vi "Lab Panel V4.83.vi"() -> ()   [LabVIEW 2013] (continued)
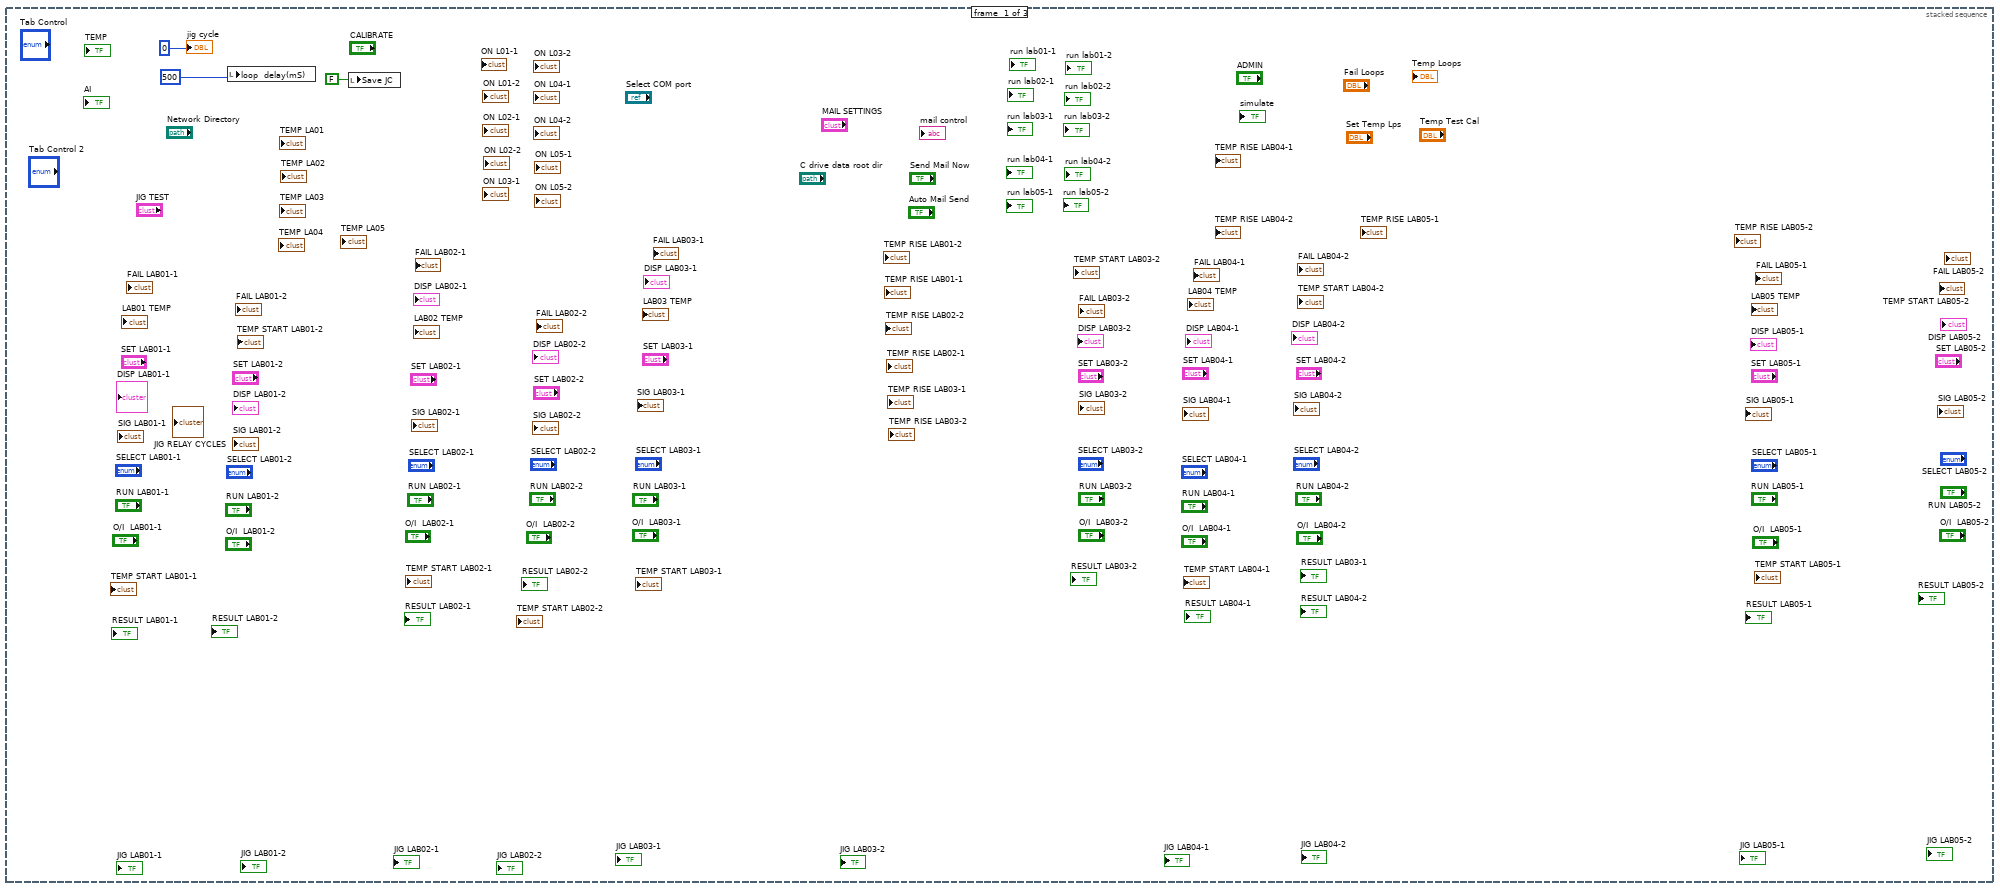
[diagram p2: hidden frame]
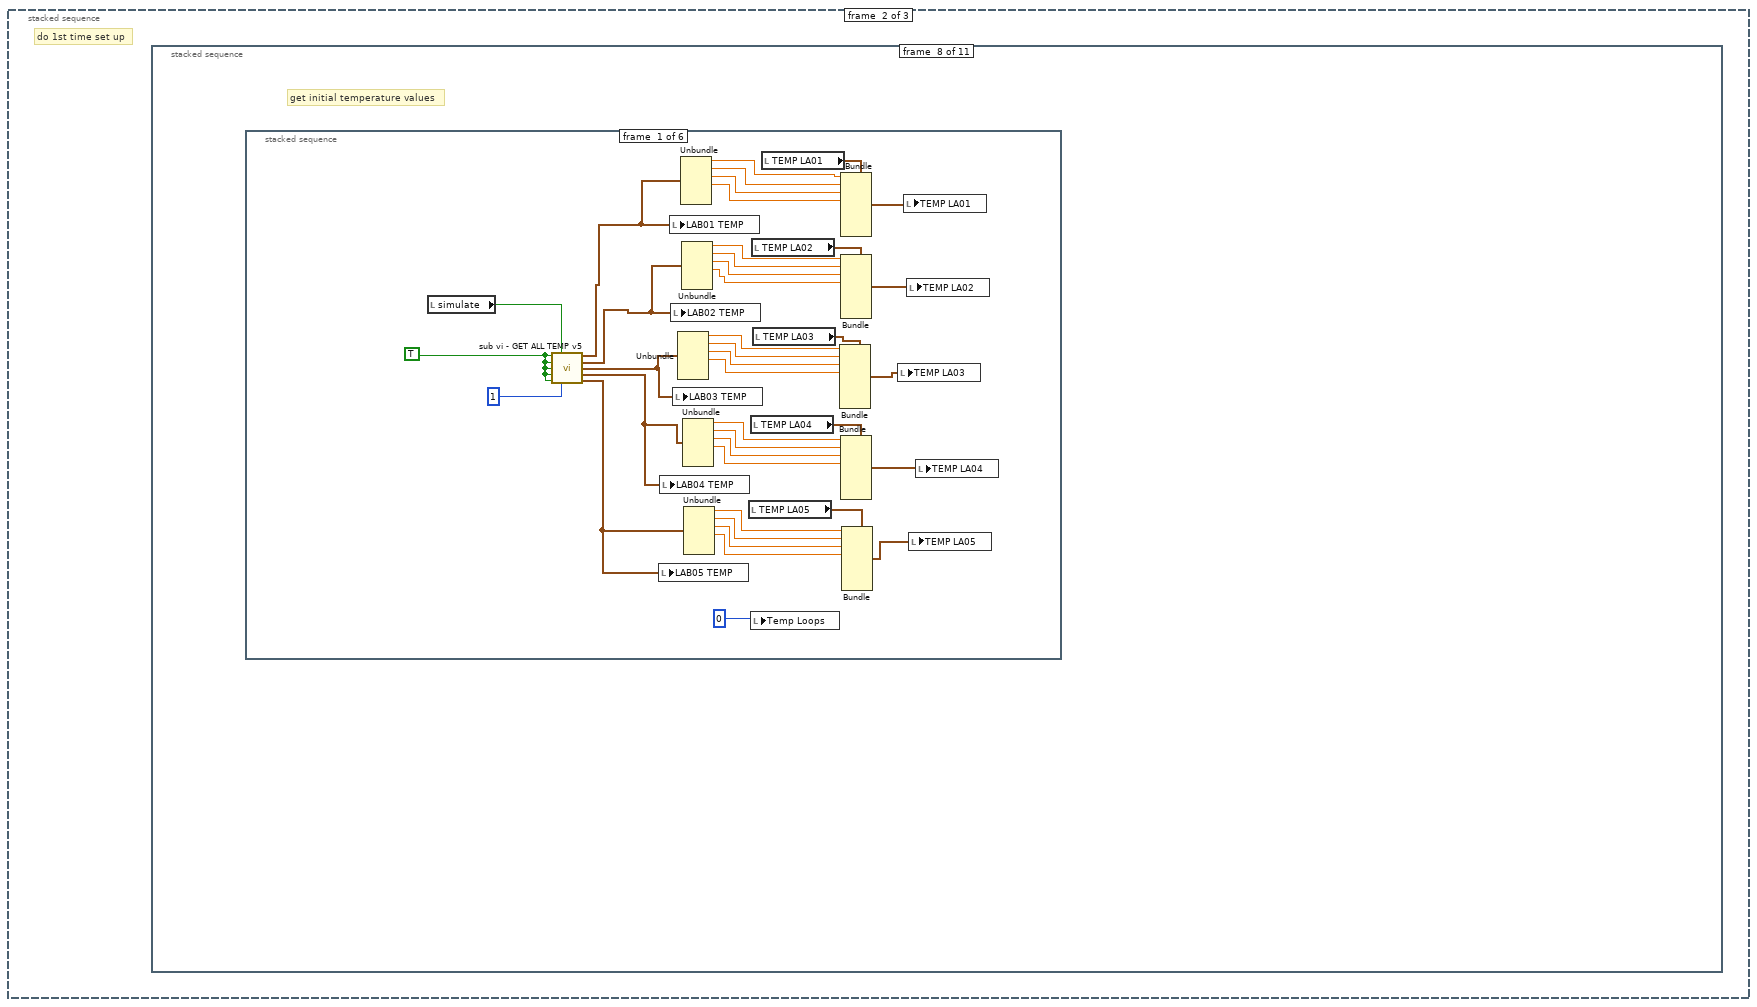
[diagram p3: hidden frame]
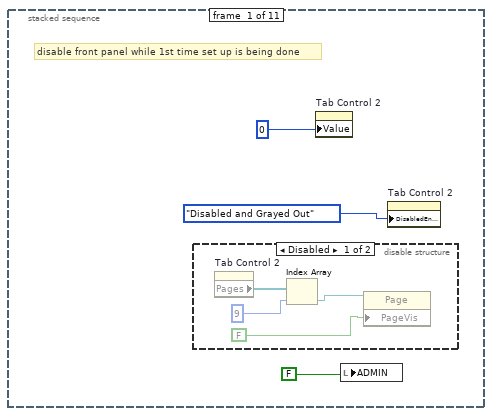
[diagram p4: hidden frame]
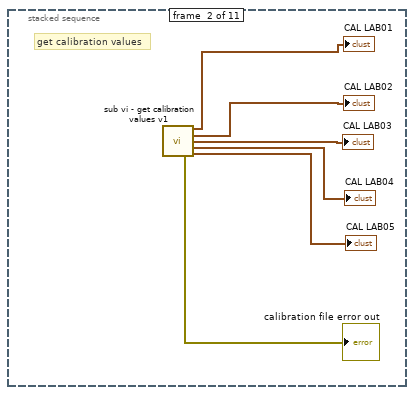
[diagram p6: hidden frame]
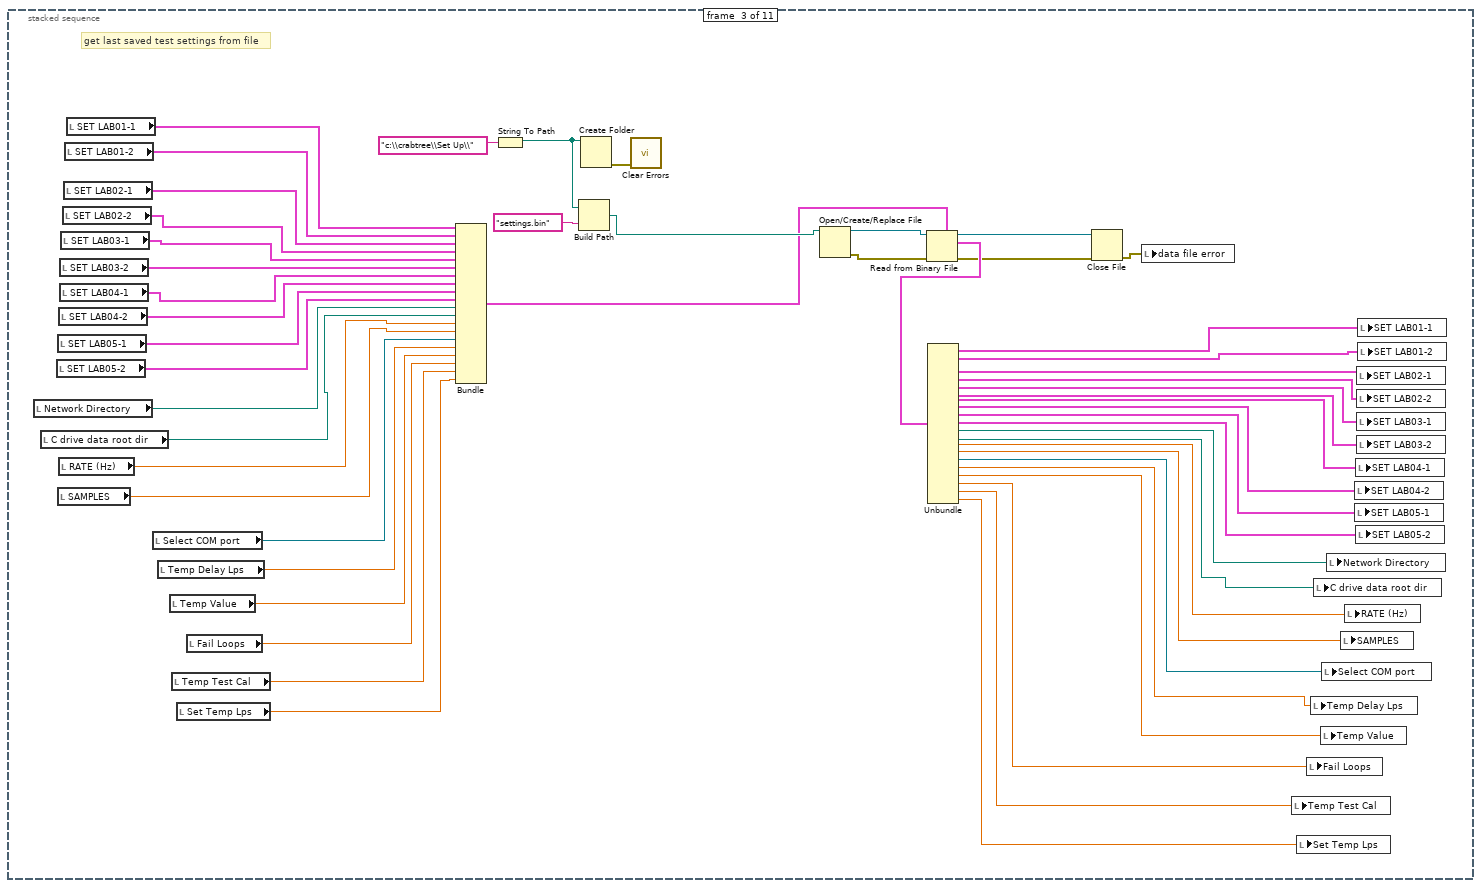
[diagram p7: hidden frame]
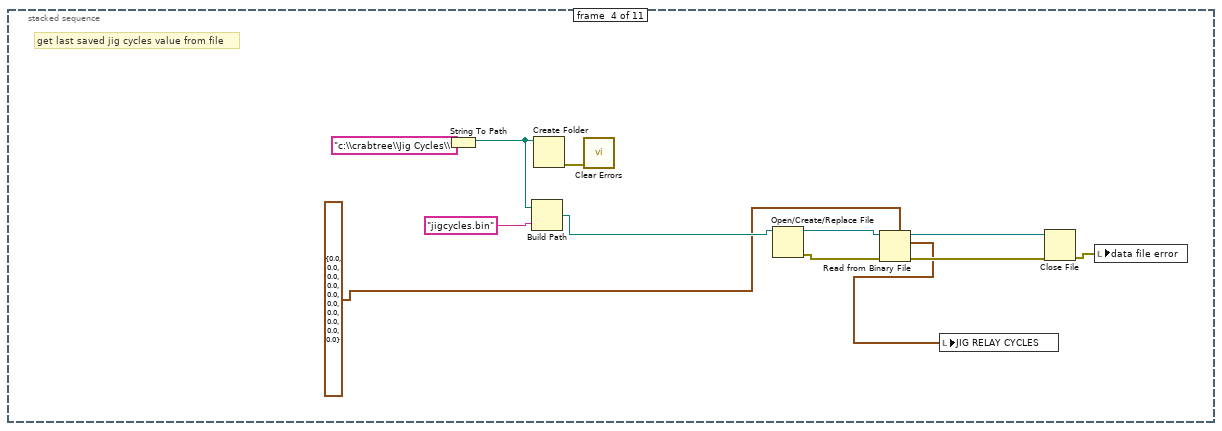
[diagram p8: hidden frame]
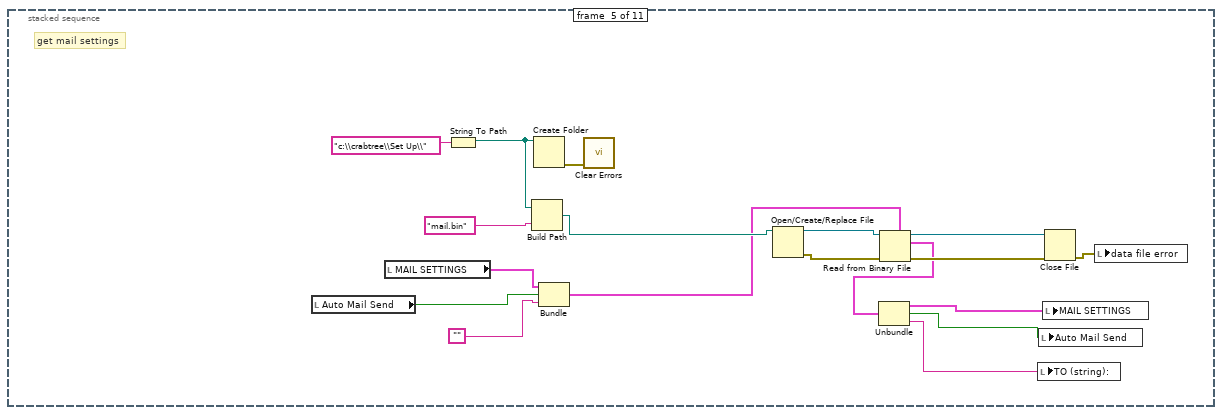
[diagram p9: hidden frame]
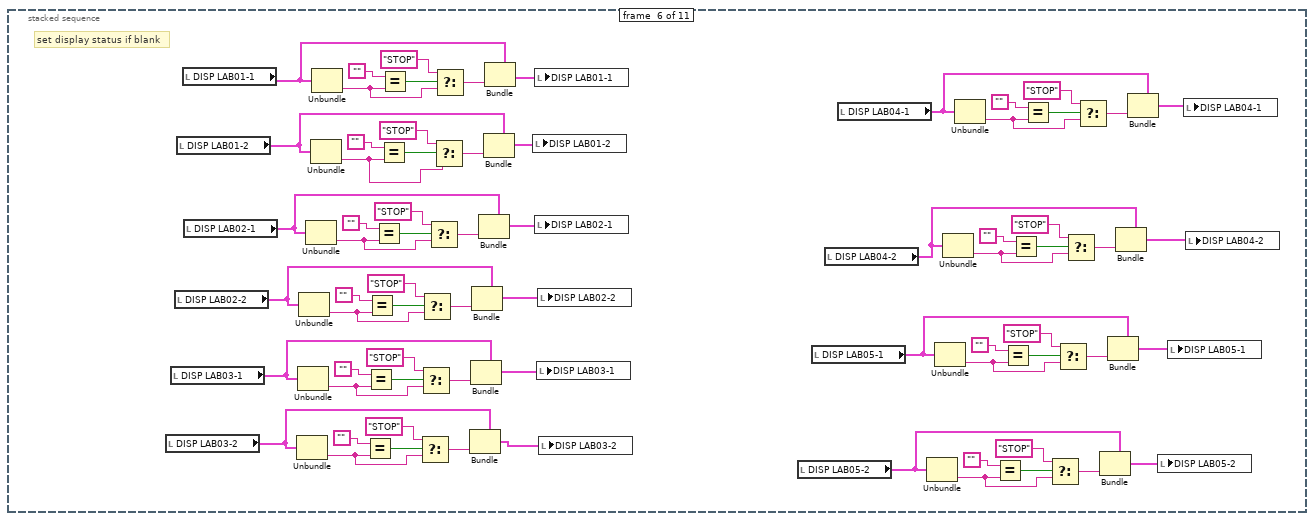
[diagram p10: hidden frame]
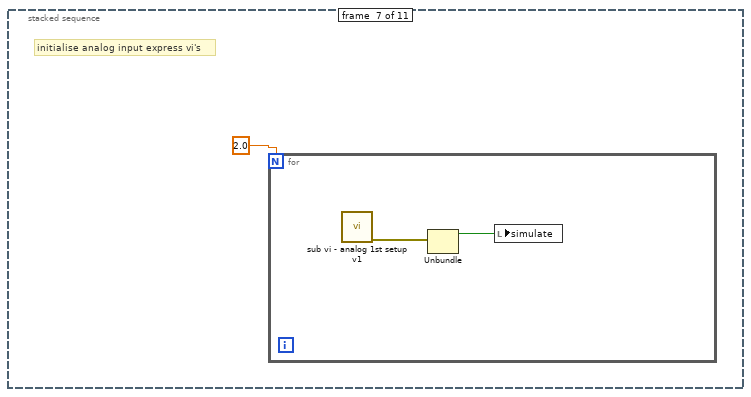
[diagram p11: hidden frame]
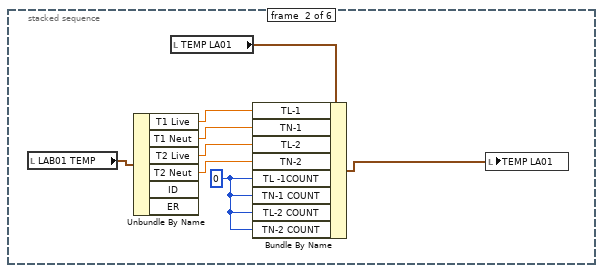
[diagram p12: hidden frame]
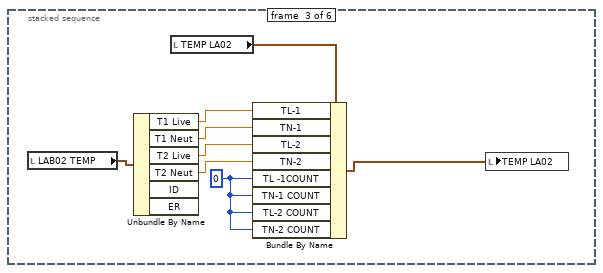
[diagram p13: hidden frame]
                              tunnel: w4562 -> [w4566 _]
                              tunnel: w4563 -> [_ w4567]
                              frame False {
                              }
                              frame True {
                                n2699 = Concatenate Strings("LA03-1 ", w4567) -> (w4570:string)
                                n2700 = One Button Dialog(message=w4570) -> ()  [unwired: 1 in, 1 out]
                              }
                            }
                          }
                          frame #5 {
                            n2701 = Greater?(x=w4571, y=w4575) -> (0:w4574:bool)
                            n2702 = case shown="True" w4574 {
                              tunnel: [w4576 0] -> w4572
                              tunnel: w4571 -> [w4576 _]
                              tunnel: w4573 -> [_ w4577]
                              frame False {
                              }
                              frame True {
                                n2703 = Concatenate Strings("LA03-2 ", w4577) -> (w4580:string)
                                n2704 = One Button Dialog(message=w4580) -> ()  [unwired: 1 in, 1 out]
                              }
                            }
                          }
                          frame #6 {
                            n2705 = Greater?(x=w4582, y=w4585) -> (0:w4584:bool)
                            n2706 = case shown="True" w4584 {
                              tunnel: [w4586 0] -> w4581
                              tunnel: w4582 -> [w4586 _]
                              tunnel: w4583 -> [_ w4587]
                              frame False {
                              }
                              frame True {
                                n2707 = Concatenate Strings("LA04-1 ", w4587) -> (w4590:string)
                                n2708 = One Button Dialog(message=w4590) -> ()  [unwired: 1 in, 1 out]
                              }
                            }
                          }
                          frame #7 {
                            n2709 = Greater?(x=w4592, y=w4595) -> (0:w4594:bool)
                            n2710 = case shown="True" w4594 {
                              tunnel: [w4596 0] -> w4591
                              tunnel: w4592 -> [w4596 _]
                              tunnel: w4593 -> [_ w4597]
                              frame False {
                              }
                              frame True {
                                n2711 = Concatenate Strings("LA04-2 ", w4597) -> (w4600:string)
                                n2712 = One Button Dialog(message=w4600) -> ()  [unwired: 1 in, 1 out]
                              }
                            }
                          }
                          frame #8 {
                            n2713 = Greater?(x=w4602, y=w4605) -> (0:w4604:bool)
                            n2714 = case shown="True" w4604 {
                              tunnel: [w4606 0] -> w4601
                              tunnel: w4602 -> [w4606 _]
                              tunnel: w4603 -> [_ w4607]
                              frame False {
                              }
                              frame True {
                                n2715 = Concatenate Strings("LA05-1 ", w4607) -> (w4610:string)
                                n2716 = One Button Dialog(message=w4610) -> ()  [unwired: 1 in, 1 out]
                              }
                            }
                          }
                          frame #9 {
                            n2717 = Greater?(x=w4612, y=w4615) -> (0:w4614:bool)
                            n2718 = case shown="True" w4614 {
                              tunnel: [w4616 0] -> w4611
                              tunnel: w4612 -> [w4616 _]
                              tunnel: w4613 -> [_ w4617]
                              frame False {
                              }
                              frame True {
                                n2719 = Concatenate Strings("LA05-2 ", w4617) -> (w4620:string)
                                n2720 = One Button Dialog(message=w4620) -> ()  [unwired: 1 in, 1 out]
                              }
                            }
                          }
                        }
                        n2721 = Bundle By Name(cluster=w4519, "LAB01-1"=w4517, "LAB01-2"=w4515, "LAB02-1"=w4512, "LAB02-2"=w4509, "LAB03-1"=w4507, "LAB03-2"=w4506, "LAB04-1"=w4503, "LAB04-2"=w4501, "LAB05-1"=w4499, "LAB05-2"=w4497) -> (w4518:T7)
                        n2722 = local write "JIG RELAY CYCLES"(w4518) -> ()
                      }
                    }
                  }
                }
              }
            }
          }
          frame #19 {
            # "get temperature values"
            n2723 = local read "simulate"() -> (w4625:bool)
            n2724 = local read "Temp Test Cal"() -> (w4622:dbl)
            n2725 = stacked-sequence {
              tunnel: w4625 -> [_ w4676 w4705 w4729 w4753 w4777]
              tunnel: T9 {"1  (A) cal"=1.0, "1 (V) cal"=1.0, "1 (PF) cal"=1.0, "1 (TL) cal"=1.0, "1 (TN) cal"=1.0, "2 (A) cal"=1.0, "2 (V) cal"=1.0, "2 (PF) cal"=1.0, "2 (TL) cal"=1.0, "2 (TN) cal"=1.0} ("CAL LAB01") -> [_ w4675 w4704 w4728 w4752 w4776]
              tunnel: w4623 -> [_ w4673 _ _ _ _]
              tunnel: w4622 -> [_ w4671 _ _ _ _]
              tunnel: w4621 -> [_ _ _ _ _ _]
              frame #0 {
                n2726 = local read "Select COM port"() -> (w4630:refnum<visa-resource-name>)
                "COM port" <- w4630
                n2727 = local read "jig cycle"() -> (w4631:dbl)
                n2728 = local read "on loops"() -> (w4633:dbl)
                n2729 = global write "Global 1.vi" "tmp dly lps"("Temp Delay Lps") -> ()
                n2730 = global write "Global 1.vi" "dly value"("Temp Value") -> ()
                n2731 = Add(x=w4633, y=3) -> (x+y=w4634:dbl)
                n2732 = global write "Global 1.vi" "COM port"(w4630) -> ()
                n2733 = Equal?(x=w4631, y=w4634) -> (x = y?=w4627:bool)
                n2734 = local read "Temp Loops"() -> (w4626:dbl)
                n2735 = case shown="True" w4627 {
                  tunnel: w4626 -> [_ w4636]
                  frame False {
                  }
                  frame True {
                    n2736 = stacked-sequence {
                      tunnel: w4636 -> [w4639 w4667]
                      frame #0 {
                        n2737 = local read "simulate"() -> (w4637:bool)
                        n2738 = case shown="5" w4639 {
                          tunnel: 1.0 -> [_ w4644 w4646 w4652 w4656 w4661]
                          tunnel: w4637 -> [_ w4640 w4645 w4650 w4657 w4660]
                          frame 0, Default {
                          }
                          frame 1 {
                            w4642 = FALSE
                            n2739 = call "sub vi - GET ALL TEMP v5.vi"("LA01-EN"=TRUE, "simulate"=w4640, "LA02-EN"=w4642, "LA03-EN"=w4642, "LA04-EN"=w4642, "LA05-EN"=w4642, "Gen Cal Value"=w4644) -> ("LA01 TEMP"=w4641:T22)  [unwired: 3 in, 5 out]
                            n2740 = local write "LAB01 TEMP"(w4641) -> ()
                          }
                          frame 2 {
                            w4647 = FALSE
                            n2741 = call "sub vi - GET ALL TEMP v5.vi"("LA01-EN"=w4647, "simulate"=w4645, "LA02-EN"=TRUE, "LA03-EN"=w4647, "LA04-EN"=w4647, "LA05-EN"=w4647, "Gen Cal Value"=w4646) -> ("LA02 TEMP"=w4649:T22)  [unwired: 3 in, 5 out]
                            n2742 = local write "LAB02 TEMP"(w4649) -> ()
                          }
                          frame 3 {
                            w4653 = FALSE
                            n2743 = call "sub vi - GET ALL TEMP v5.vi"("LA01-EN"=w4653, "simulate"=w4650, "LA02-EN"=w4653, "LA03-EN"=TRUE, "LA04-EN"=w4653, "LA05-EN"=w4653, "Gen Cal Value"=w4652) -> ("LA03 TEMP"=w4651:T22)  [unwired: 3 in, 5 out]
                            n2744 = local write "LAB03 TEMP"(w4651) -> ()
                          }
                          frame 4 {
                            w4658 = FALSE
                            n2745 = call "sub vi - GET ALL TEMP v5.vi"("LA01-EN"=w4658, "simulate"=w4657, "LA02-EN"=w4658, "LA03-EN"=w4658, "LA04-EN"=TRUE, "LA05-EN"=w4658, "Gen Cal Value"=w4656) -> ("LA04 TEMP"=w4655:T22)  [unwired: 3 in, 5 out]
                            n2746 = local write "LAB04 TEMP"(w4655) -> ()
                          }
                          frame 5 {
                            w4663 = FALSE
                            n2747 = call "sub vi - GET ALL TEMP v5.vi"("LA01-EN"=w4663, "simulate"=w4660, "LA02-EN"=w4663, "LA03-EN"=w4663, "LA04-EN"=w4663, "LA05-EN"=TRUE, "Gen Cal Value"=w4661) -> ("LA05 TEMP"=w4662:T22)  [unwired: 3 in, 5 out]
                            n2748 = local write "LAB05 TEMP"(w4662) -> ()
                          }
                        }
                      }
                      frame #1 {
                        n2749 = Greater Or Equal?(x=w4667, y=5) -> (x >= y?=w4665:bool)
                        n2750 = case shown="True" w4665 {
                          frame False {
                          }
                          frame True {
                            n2751 = local write "Temp Loops"(0) -> ()
                          }
                        }
                      }
                    }
                    n2752 = local write "TEMP"(TRUE) -> ()
                  }
                }
              }
              frame #1 {
                n2753 = case shown="False" w4676 {
                  tunnel: [w4702 w4703] -> w4694
                  tunnel: w4675 -> [_ w4703]
                  frame False {
                    n2754 = local read "CAL LAB01"() -> (w4702:T9)
                  }
                  frame True {
                  }
                }
                n2755 = local read "LAB01 TEMP"() -> (w4682:T13)
                n2756 = local read "TEMP LA01"() -> (w4683:T8)
                n2757 = call "sub vi - temperature delay v2.vi"("temp values IN"=w4683, "temp signals"=w4682) -> ("T2-N"=w4678:dbl, "T2-L"=w4679:dbl, "T1-N"=w4680:dbl, "T1-L"=w4681:dbl, "temp values OUT"=w4677:T39)  [unwired: 5 in]
                n2758 = Unbundle By Name(w4694) -> ("1 (TL) cal"=w4687:dbl, "1 (TN) cal"=w4686:dbl, "2 (TL) cal"=w4685:dbl, "2 (TN) cal"=w4684:dbl)  [unwired: 6 out]
                n2759 = local write "TEMP LA01"(w4677) -> ()
                n2760 = Multiply(x=w4681, y=w4687) -> (x*y=w4674:dbl)
                n2761 = Multiply(x=w4680, y=w4686) -> (x*y=w4670:dbl)
                n2762 = Multiply(x=w4679, y=w4685) -> (x*y=w4689:dbl)
                n2763 = Multiply(x=w4678, y=w4684) -> (x*y=w4688:dbl)
                n2764 = case shown="True" w4673 {
                  tunnel: w4674 -> [w4696 w4701]
                  tunnel: w4671 -> [_ w4699]
                  tunnel: [w4696 w4700] -> w4672
                  tunnel: w4670 -> [w4695 w4698]
                  tunnel: [w4695 w4697] -> w4669
                  frame False {
                  }
                  frame True {
                    n2765 = Multiply(x=w4699, y=w4698) -> (x*y=w4697:dbl)
                    n2766 = Multiply(x=w4699, y=w4701) -> (x*y=w4700:dbl)
                  }
                }
                n2767 = local read "SIG LAB01-2"() -> (w4691:T2)
                n2768 = local read "SIG LAB01-1"() -> (w4693:T2)
                n2769 = Bundle By Name(cluster=w4693, "Tmp Live"=w4672, "Tmp Neut"=w4669) -> (w4692:T2)
                n2770 = Bundle By Name(cluster=w4691, "Tmp Live"=w4689, "Tmp Neut"=w4688) -> (w4690:T2)
                n2771 = local write "SIG LAB01-1"(w4692) -> ()
                n2772 = local write "SIG LAB01-2"(w4690) -> ()
              }
              frame #2 {
                n2773 = case shown="True" w4705 {
                  tunnel: [w4726 w4727] -> w4725
                  tunnel: w4704 -> [_ w4727]
                  frame False {
                    n2774 = local read "CAL LAB02"() -> (w4726:T10)
                  }
                  frame True {
                  }
                }
                n2775 = local read "LAB02 TEMP"() -> (w4712:T13)
                n2776 = local read "TEMP LA02"() -> (w4711:T8)
                n2777 = call "sub vi - temperature delay v2.vi"("temp values IN"=w4711, "temp signals"=w4712) -> ("T2-N"=w4706:dbl, "T2-L"=w4707:dbl, "T1-N"=w4708:dbl, "T1-L"=w4709:dbl, "temp values OUT"=w4710:T39)  [unwired: 5 in]
                n2778 = Unbundle By Name(w4725) -> ("1 (TL) cal"=w4716:dbl, "1 (TN) cal"=w4715:dbl, "2 (TL) cal"=w4714:dbl, "2 (TN) cal"=w4713:dbl)  [unwired: 6 out]
                n2779 = local write "TEMP LA02"(w4710) -> ()
                n2780 = Multiply(x=w4709, y=w4716) -> (x*y=w4722:dbl)
                n2781 = Multiply(x=w4708, y=w4715) -> (x*y=w4721:dbl)
                n2782 = Multiply(x=w4707, y=w4714) -> (x*y=w4718:dbl)
                n2783 = Multiply(x=w4706, y=w4713) -> (x*y=w4717:dbl)
                n2784 = local read "SIG LAB02-2"() -> (w4720:T2)
                n2785 = local read "SIG LAB02-1"() -> (w4724:T2)
                n2786 = Bundle By Name(cluster=w4724, "Tmp Live"=w4722, "Tmp Neut"=w4721) -> (w4723:T2)
                n2787 = Bundle By Name(cluster=w4720, "Tmp Live"=w4718, "Tmp Neut"=w4717) -> (w4719:T2)
                n2788 = local write "SIG LAB02-1"(w4723) -> ()
                n2789 = local write "SIG LAB02-2"(w4719) -> ()
              }
              frame #3 {
                n2790 = case shown="False" w4729 {
                  tunnel: [w4750 w4751] -> w4749
                  tunnel: w4728 -> [_ w4751]
                  frame False {
                    n2791 = local read "CAL LAB03"() -> (w4750:T9)
                  }
                  frame True {
                  }
                }
                n2792 = local read "TEMP LA03"() -> (w4735:T8)
                n2793 = local read "LAB03 TEMP"() -> (w4736:T13)
                n2794 = call "sub vi - temperature delay v2.vi"("temp values IN"=w4735, "temp signals"=w4736) -> ("T2-N"=w4730:dbl, "T2-L"=w4731:dbl, "T1-N"=w4732:dbl, "T1-L"=w4733:dbl, "temp values OUT"=w4734:T39)  [unwired: 5 in]
                n2795 = Unbundle By Name(w4749) -> ("1 (TL) cal"=w4740:dbl, "1 (TN) cal"=w4739:dbl, "2 (TL) cal"=w4738:dbl, "2 (TN) cal"=w4737:dbl)  [unwired: 6 out]
                n2796 = local write "TEMP LA03"(w4734) -> ()
                n2797 = Multiply(x=w4733, y=w4740) -> (x*y=w4746:dbl)
                n2798 = Multiply(x=w4732, y=w4739) -> (x*y=w4745:dbl)
                n2799 = Multiply(x=w4731, y=w4738) -> (x*y=w4742:dbl)
                n2800 = Multiply(x=w4730, y=w4737) -> (x*y=w4741:dbl)
                n2801 = local read "SIG LAB03-2"() -> (w4744:T2)
                n2802 = local read "SIG LAB03-1"() -> (w4748:T2)
                n2803 = Bundle By Name(cluster=w4748, "Tmp Live"=w4746, "Tmp Neut"=w4745) -> (w4747:T2)
                n2804 = Bundle By Name(cluster=w4744, "Tmp Live"=w4742, "Tmp Neut"=w4741) -> (w4743:T2)
                n2805 = local write "SIG LAB03-1"(w4747) -> ()
                n2806 = local write "SIG LAB03-2"(w4743) -> ()
              }
              frame #4 {
                n2807 = case shown="False" w4753 {
                  tunnel: [w4774 w4775] -> w4773
                  tunnel: w4752 -> [_ w4775]
                  frame False {
                    n2808 = local read "CAL LAB04"() -> (w4774:T9)
                  }
                  frame True {
                  }
                }
                n2809 = local read "LAB04 TEMP"() -> (w4759:T13)
                n2810 = local read "TEMP LA04"() -> (w4760:T8)
                n2811 = call "sub vi - temperature delay v2.vi"("temp values IN"=w4760, "temp signals"=w4759) -> ("T2-N"=w4754:dbl, "T2-L"=w4755:dbl, "T1-N"=w4756:dbl, "T1-L"=w4757:dbl, "temp values OUT"=w4758:T39)  [unwired: 5 in]
                n2812 = Unbundle By Name(w4773) -> ("1 (TL) cal"=w4764:dbl, "1 (TN) cal"=w4763:dbl, "2 (TL) cal"=w4762:dbl, "2 (TN) cal"=w4761:dbl)  [unwired: 6 out]
                n2813 = local write "TEMP LA04"(w4758) -> ()
                n2814 = Multiply(x=w4757, y=w4764) -> (x*y=w4770:dbl)
                n2815 = Multiply(x=w4756, y=w4763) -> (x*y=w4769:dbl)
                n2816 = Multiply(x=w4755, y=w4762) -> (x*y=w4766:dbl)
                n2817 = Multiply(x=w4754, y=w4761) -> (x*y=w4765:dbl)
                n2818 = local read "SIG LAB04-2"() -> (w4768:T2)
                n2819 = local read "SIG LAB04-1"() -> (w4772:T2)
                n2820 = Bundle By Name(cluster=w4772, "Tmp Live"=w4770, "Tmp Neut"=w4769) -> (w4771:T2)
                n2821 = Bundle By Name(cluster=w4768, "Tmp Live"=w4766, "Tmp Neut"=w4765) -> (w4767:T2)
                n2822 = local write "SIG LAB04-1"(w4771) -> ()
                n2823 = local write "SIG LAB04-2"(w4767) -> ()
              }
              frame #5 {
                n2824 = case shown="False" w4777 {
                  tunnel: [w4798 w4799] -> w4797
                  tunnel: w4776 -> [_ w4799]
                  frame False {
                    n2825 = local read "CAL LAB05"() -> (w4798:T9)
                  }
                  frame True {
                  }
                }
                n2826 = local read "LAB05 TEMP"() -> (w4783:T13)
                n2827 = local read "TEMP LA05"() -> (w4784:T8)
                n2828 = call "sub vi - temperature delay v2.vi"("temp values IN"=w4784, "temp signals"=w4783) -> ("T2-N"=w4779:dbl, "T2-L"=w4780:dbl, "T1-N"=w4781:dbl, "T1-L"=w4782:dbl, "temp values OUT"=w4778:T39)  [unwired: 5 in]
                n2829 = local write "TEMP LA05"(w4778) -> ()
                n2830 = Unbundle By Name(w4797) -> ("1 (TL) cal"=w4785:dbl, "1 (TN) cal"=w4788:dbl, "2 (TL) cal"=w4787:dbl, "2 (TN) cal"=w4786:dbl)  [unwired: 6 out]
                n2831 = Multiply(x=w4782, y=w4785) -> (x*y=w4794:dbl)
                n2832 = Multiply(x=w4781, y=w4788) -> (x*y=w4793:dbl)
                n2833 = Multiply(x=w4780, y=w4787) -> (x*y=w4790:dbl)
                n2834 = Multiply(x=w4779, y=w4786) -> (x*y=w4789:dbl)
                n2835 = local read "SIG LAB05-2"() -> (w4792:T2)
                n2836 = local read "SIG LAB05-1"() -> (w4796:T2)
                n2837 = Bundle By Name(cluster=w4796, "Tmp Live"=w4794, "Tmp Neut"=w4793) -> (w4795:T2)
                n2838 = Bundle By Name(cluster=w4792, "Tmp Live"=w4790, "Tmp Neut"=w4789) -> (w4791:T2)
                n2839 = local write "SIG LAB05-1"(w4795) -> ()
                n2840 = local write "SIG LAB05-2"(w4791) -> ()
              }
            }
          }
          frame #20 {
            # "write data to display panel and end all programs running"
            n2841 = local read "O/I  LAB05-2"() -> (w4840:bool)
            n2842 = local read "O/I  LAB05-1"() -> (w4841:bool)
            n2843 = local read "O/I  LAB03-2"() -> (w4844:bool)
            n2844 = local read "O/I  LAB04-2"() -> (w4842:bool)
            n2845 = local read "O/I  LAB04-1"() -> (w4843:bool)
            n2846 = local read "O/I  LAB03-1"() -> (w4845:bool)
            n2847 = local read "O/I  LAB01-2"() -> (w4848:bool)
            n2848 = local read "O/I  LAB01-1"() -> (w4849:bool)
            n2849 = local read "O/I  LAB02-1"() -> (w4847:bool)
            n2850 = local read "O/I  LAB02-2"() -> (w4846:bool)
            n2851 = Quit LabVIEW(quit? (T)="stop all") -> ()
            n2852 = global write "Global display 1.vi" "5-2 O/F"(w4840) -> ()
            n2853 = global write "Global display 1.vi" "5-1 O/F"(w4841) -> ()
            n2854 = global write "Global display 1.vi" "4-1 O/F"(w4843) -> ()
            n2855 = global write "Global display 1.vi" "4-2 O/F"(w4842) -> ()
            n2856 = global write "Global display 1.vi" "3-2 O/F"(w4844) -> ()
            n2857 = global write "Global display 1.vi" "3-1 O/F"(w4845) -> ()
            n2858 = global write "Global display 1.vi" "2-2 O/F"(w4846) -> ()
            n2859 = global write "Global display 1.vi" "2-1 O/F"(w4847) -> ()
            n2860 = global write "Global display 1.vi" "1-2 O/F"(w4848) -> ()
            n2861 = global write "Global display 1.vi" "1-1 O/F"(w4849) -> ()
            n2862 = global write "Global display 1.vi" "stop disp"("stop all") -> ()
            n2863 = local read "RUN LAB05-2"() -> (w4830:bool)
            n2864 = local read "RUN LAB04-1"() -> (w4833:bool)
            n2865 = local read "RUN LAB04-2"() -> (w4832:bool)
            n2866 = local read "RUN LAB05-1"() -> (w4831:bool)
            n2867 = local read "RUN LAB03-2"() -> (w4834:bool)
            n2868 = local read "RUN LAB02-1"() -> (w4837:bool)
            n2869 = local read "RUN LAB03-1"() -> (w4835:bool)
            n2870 = local read "RUN LAB01-2"() -> (w4838:bool)
            n2871 = local read "RUN LAB02-2"() -> (w4836:bool)
            n2872 = local read "RUN LAB01-1"() -> (w4839:bool)
            n2873 = global write "Global display 1.vi" "5-2 R/S"(w4830) -> ()
            n2874 = global write "Global display 1.vi" "5-1 R/S"(w4831) -> ()
            n2875 = global write "Global display 1.vi" "4-2 R/S"(w4832) -> ()
            n2876 = global write "Global display 1.vi" "4-1 R/S"(w4833) -> ()
            n2877 = global write "Global display 1.vi" "3-2 R/S"(w4834) -> ()
            n2878 = global write "Global display 1.vi" "1-2 R/S"(w4838) -> ()
            n2879 = global write "Global display 1.vi" "2-1 R/S"(w4837) -> ()
            n2880 = global write "Global display 1.vi" "3-1 R/S"(w4835) -> ()
            n2881 = global write "Global display 1.vi" "2-2 R/S"(w4836) -> ()
            n2882 = global write "Global display 1.vi" "1-1 R/S"(w4839) -> ()
            n2883 = local read "DISP LAB04-2"() -> (w4822:T4)
            n2884 = local read "DISP LAB05-1"() -> (w4821:T4)
            n2885 = local read "DISP LAB04-1"() -> (w4823:T4)
            n2886 = local read "DISP LAB05-2"() -> (w4820:T4)
            n2887 = local read "DISP LAB03-1"() -> (w4825:T4)
            n2888 = local read "DISP LAB03-2"() -> (w4824:T4)
            n2889 = local read "DISP LAB01-2"() -> (w4828:T4)
            n2890 = local read "DISP LAB02-1"() -> (w4827:T4)
            n2891 = local read "DISP LAB02-2"() -> (w4826:T4)
            n2892 = local read "DISP LAB01-1"() -> (w4829:T4)
            n2893 = global write "Global display 2.vi" "DISP LAB05-1"(w4821) -> ()
            n2894 = global write "Global display 2.vi" "DISP LAB05-2"(w4820) -> ()
            n2895 = global write "Global display 2.vi" "DISP LAB04-2"(w4822) -> ()
            n2896 = global write "Global display 2.vi" "DISP LAB02-1"(w4827) -> ()
            n2897 = global write "Global display 2.vi" "DISP LAB02-2"(w4826) -> ()
            n2898 = global write "Global display 2.vi" "DISP LAB04-1"(w4823) -> ()
            n2899 = global write "Global display 2.vi" "DISP LAB01-2"(w4828) -> ()
            n2900 = global write "Global display 2.vi" "DISP LAB01-1"(w4829) -> ()
            n2901 = global write "Global display 2.vi" "DISP LAB03-1"(w4825) -> ()
            n2902 = global write "Global display 2.vi" "DISP LAB03-2"(w4824) -> ()
            n2903 = local read "SET LAB05-2"() -> (w4810:T5)
            n2904 = local read "SET LAB05-1"() -> (w4811:T5)
            n2905 = local read "SET LAB04-1"() -> (w4813:T5)
            n2906 = local read "SET LAB04-2"() -> (w4812:T5)
            n2907 = local read "SET LAB03-1"() -> (w4815:T5)
            n2908 = local read "SET LAB03-2"() -> (w4814:T5)
            n2909 = local read "SET LAB02-2"() -> (w4816:T5)
            n2910 = local read "SET LAB01-2"() -> (w4818:T5)
            n2911 = local read "SET LAB02-1"() -> (w4817:T5)
            n2912 = local read "SET LAB01-1"() -> (w4819:T5)
            n2913 = global write "Global display 2.vi" "SET LAB01-1"(w4810) -> ()
            n2914 = global write "Global display 2.vi" "SET LAB01-1"(w4811) -> ()
            n2915 = global write "Global display 2.vi" "SET LAB01-1"(w4813) -> ()
            n2916 = global write "Global display 2.vi" "SET LAB01-1"(w4812) -> ()
            n2917 = global write "Global display 2.vi" "SET LAB01-1"(w4814) -> ()
            n2918 = global write "Global display 2.vi" "SET LAB01-1"(w4816) -> ()
            n2919 = global write "Global display 2.vi" "SET LAB01-1"(w4815) -> ()
            n2920 = global write "Global display 2.vi" "SET LAB01-1"(w4818) -> ()
            n2921 = global write "Global display 2.vi" "SET LAB01-1"(w4819) -> ()
            n2922 = global write "Global display 2.vi" "SET LAB01-1"(w4817) -> ()
            n2923 = local read "RESULT LAB01-1"() -> (w4809:bool)
            n2924 = local read "RESULT LAB03-2"() -> (w4804:bool)
            n2925 = local read "RESULT LAB04-1"() -> (w4803:bool)
            n2926 = local read "RESULT LAB04-2"() -> (w4802:bool)
            n2927 = local read "RESULT LAB02-2"() -> (w4806:bool)
            n2928 = local read "RESULT LAB01-2"() -> (w4808:bool)
            n2929 = local read "RESULT LAB02-1"() -> (w4807:bool)
            n2930 = local read "RESULT LAB03-1"() -> (w4805:bool)
            n2931 = local read "RESULT LAB05-1"() -> (w4801:bool)
            n2932 = local read "RESULT LAB05-2"() -> (w4800:bool)
            n2933 = global write "Global display 2.vi" "RESULT LAB05-1"(w4801) -> ()
            n2934 = global write "Global display 2.vi" "RESULT LAB01-2"(w4808) -> ()
            n2935 = global write "Global display 2.vi" "RESULT LAB03-2"(w4804) -> ()
            n2936 = global write "Global display 2.vi" "RESULT LAB04-1"(w4803) -> ()
            n2937 = global write "Global display 2.vi" "RESULT LAB04-2"(w4802) -> ()
            n2938 = global write "Global display 2.vi" "RESULT LAB05-2"(w4800) -> ()
            n2939 = global write "Global display 2.vi" "RESULT LAB03-1"(w4805) -> ()
            n2940 = global write "Global display 2.vi" "RESULT LAB02-1"(w4807) -> ()
            n2941 = global write "Global display 2.vi" "RESULT LAB02-2"(w4806) -> ()
            n2942 = global write "Global display 2.vi" "RESULT LAB01-1"(w4809) -> ()
          }
        }
        n2943 = node-c288() -> ()  [unwired: 1 in, 1 out]
        "loops" <- w287
      }
      n2944 = node-c288(w264) -> ()  [unwired: 1 out]
    }
  }
